vi "ActionVIOnCompile.vi"(8 "error in (no error)":errorcluster, 11 "Device Item Ref in":T2 format="%.0x") -> (0 "error out":errorcluster)   [LabVIEW 2015, in "SLSC Module Template System Explorer.lvlib"]
uses:
  SLSC Module Template System Explorer.lvlib
  <vilib>/NI Veristand/Custom Device API/Custom Device Item Ref.ctl
  Shared/SLSC Dynamic Channel.ctl
  Shared/Compiled.Settings
  Shared/Constants.vi
  <vilib>/NI Veristand/Custom Device Tools/Custom Device Utility Library/NI VeriStand - Search for Item by Name.vi
  <vilib>/NI Veristand/Custom Device API/Get Item Property (I32).vi
  <vilib>/NI Veristand/Custom Device API/Get Item Property (String).vi
  <vilib>/NI Veristand/Custom Device API/Set Item Property (Variant).vi
  <vilib>/NI Veristand/Custom Device Tools/Custom Device Utility Library/Custom Device Utility Library.lvlib
  <vilib>/NI Veristand/Custom Device API/Custom Device API.lvlib
  <vilib>/NI/NIVS Inline Async API/_Data Access System Explorer/Data Access System Explorer.lvlib
  Shared/SLSC Module Template Shared.lvlib
panel:
  out "SLSC Dynamic Commands":T1[](array[typedef])
  out "SLSC Dynamic outputs":T1[](array[typedef])
  out "SLSC Dynamic Inputs":T1[](array[typedef])
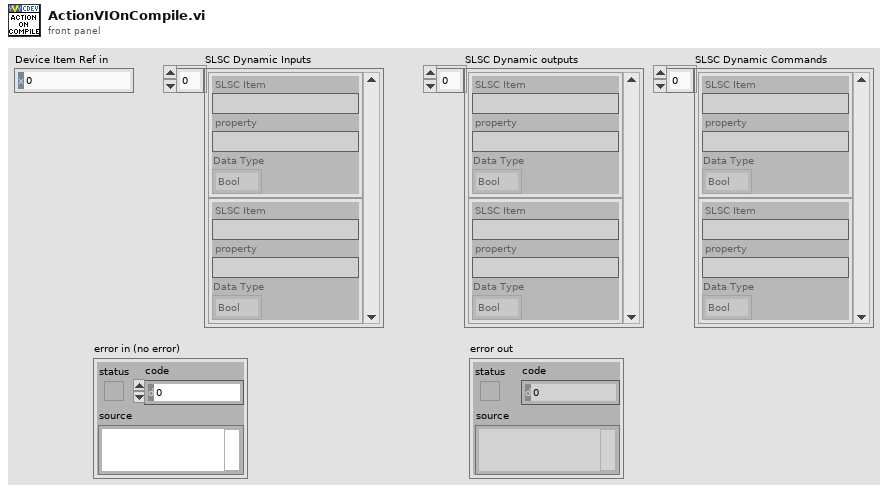
[diagram p1: front panel]
types:
  T1 = typedef "SLSC Module Template System Explorer.lvlib/SLSC Dynamic Channel.ctl" = cluster{"SLSC Item":string, "property":string, "Data Type":enum16{"Bool", "Double", "I32", "I64", "String", "U32", "U64"}}
  T2 = typedef "Custom Device API.lvlib/Custom Device Item Ref.ctl" = u64
  T3 = enum16{"Output/Write", "Input/Read", "Input/ReadWrite"}
  T4 = typedef "SLSC Module Template Shared.lvlib/Compiled.Settings" = cluster{"Name":string, "SLSC IP Address":string, "Slot #":i32, "Configuration Data":cluster{"Properties":cluster{"Boolean Properties":cluster{"property":refnum<k21>, "Value":bool, "SLSC Item":refnum<k21>}[], "Double Properties":cluster{"property":refnum<k21>, "Double Write":dbl, "SLSC Item":refnum<k21>}[], "I32 Properties":cluster{"property":refnum<k21>, "Int32 Write":i32, "SLSC Item":refnum<k21>}[], "I64 Properties":cluster{"property":refnum<k21>, "Int64 Write":i64, "SLSC Item":refnum<k21>}[], "String Properties":cluster{"property":refnum<k21>, "String Write":string, "SLSC Item":refnum<k21>}[], "U32 Properties":cluster{"property":refnum<k21>, "UInt32 Write":u32, "SLSC Item":refnum<k21>}[], "U64 Properties":cluster{"property":refnum<k21>, "UInt64 Write":u64, "SLSC Item":refnum<k21>}[]}}, "SLSC Dynamic Inputs":T1[], "SLSC Dynamic Outputs":T1[], "SLSC Dynamic Commands":T1[]}
  T5 = cluster{"Name":string, "Type":enum16{"Output/Write", "Input/Read", "Input/ReadWrite"}, "VS Refs":T2[]}
  T6 = typedef "Custom Device API.lvlib/Custom Device Item Info.ctl" = cluster{"Name":string, "Is Channel":bool, "GUID":string, "Is Waveform":bool}
  T7 = cluster{"Properties":cluster{"Boolean Properties":cluster{"property":refnum<k21>, "Value":bool, "SLSC Item":refnum<k21>}[], "Double Properties":cluster{"property":refnum<k21>, "Double Write":dbl, "SLSC Item":refnum<k21>}[], "I32 Properties":cluster{"property":refnum<k21>, "Int32 Write":i32, "SLSC Item":refnum<k21>}[], "I64 Properties":cluster{"property":refnum<k21>, "Int64 Write":i64, "SLSC Item":refnum<k21>}[], "String Properties":cluster{"property":refnum<k21>, "String Write":string, "SLSC Item":refnum<k21>}[], "U32 Properties":cluster{"property":refnum<k21>, "UInt32 Write":u32, "SLSC Item":refnum<k21>}[], "U64 Properties":cluster{"property":refnum<k21>, "UInt64 Write":u64, "SLSC Item":refnum<k21>}[]}}
  T8 = cluster{"Name":string, "Type":enum16{"Output/Write", "Input/Read", "Input/ReadWrite"}, "VS Refs":T2[]}[]
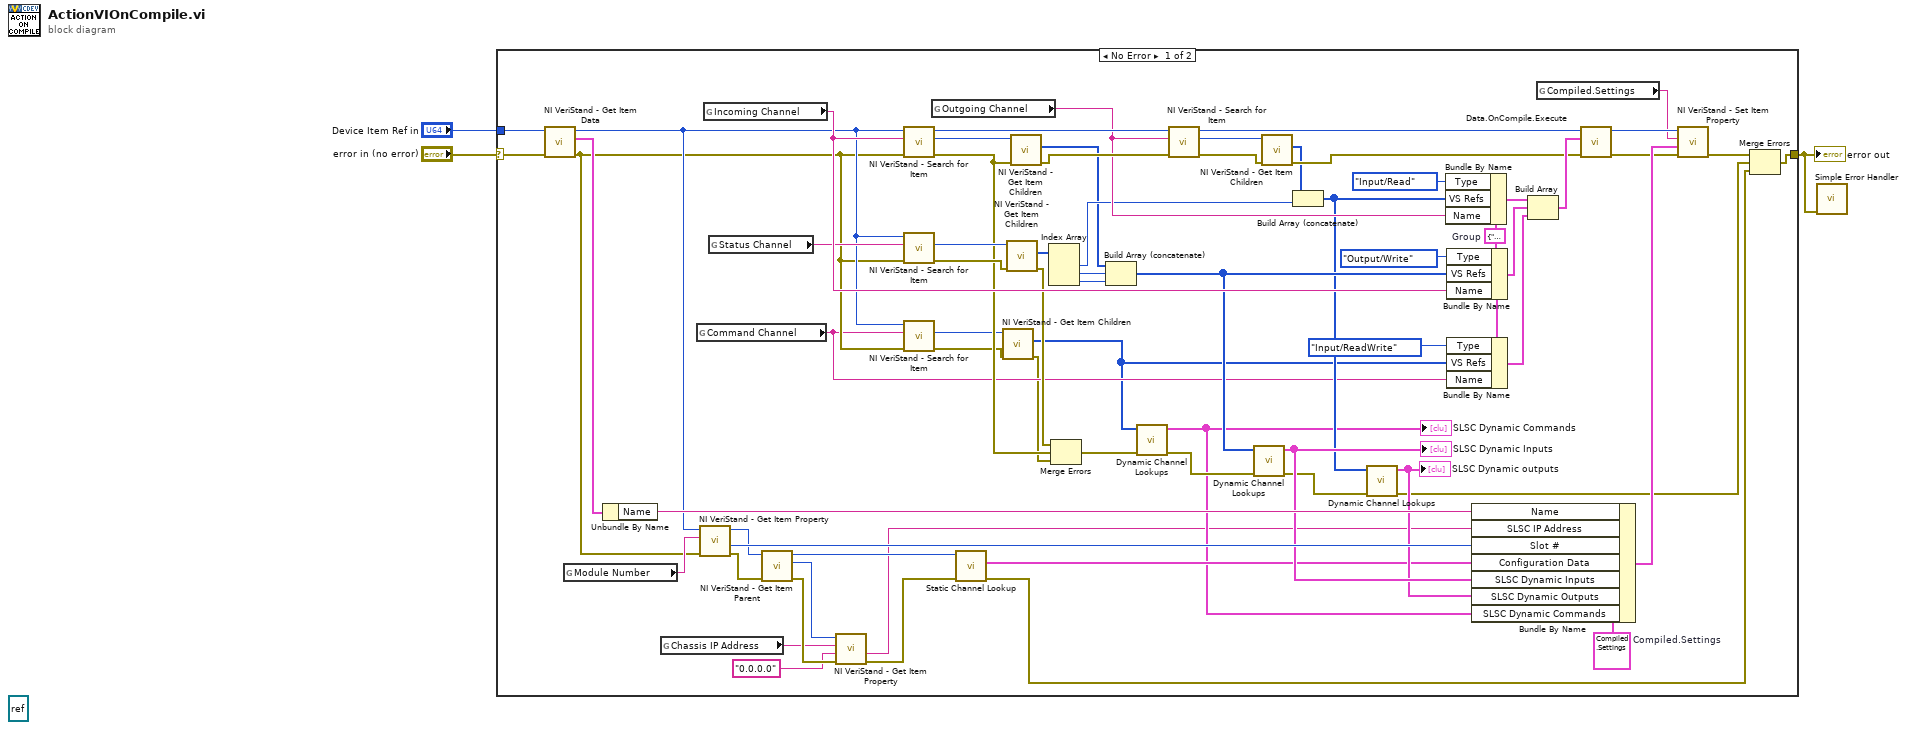
[diagram p0: block diagram]
diagram:
  (unwired) refnum<k7> refnum ("SHDocVw.IWebBrowser2")
  n1 = case shown="No Error" "error in (no error)" {
    selector: "error in (no error)" -> [w47 w72]
    tunnel: [w45 w72] -> w1
    tunnel: "Device Item Ref in" -> [w48 _]
    frame No Error {
      w38 = T4 {"Name"="", "SLSC IP Address"="", "Slot #"=0, "Configuration Data"={"Properties"={"Boolean Properties"=[], "Double Properties"=[], "I32 Properties"=[], "I64 Properties"=[], "String Properties"=[], "U32 Properties"=[], "U64 Properties"=[]}}, "SLSC Dynamic Inputs"=[], "SLSC Dynamic Outputs"=[], "SLSC Dynamic Commands"=[]}  # Compiled.Settings
      w12 = T5 {"Name"="", "Type"=enum."Output/Write", "VS Refs"=[]}  # Group
      n2 = call <vilib>:"NI VeriStand - Get Item Data.vi"("error in (no error)"=w47, "Item Ref in"=w48) -> ("error out"=w14:errorcluster, "Item Info"=w67:T6, "Item Ref out"=w15:T2)  [unwired: 6 in, 1 out]
      n3 = global read "Constants.vi" "Module Number"() -> (w50:string)
      n4 = Unbundle By Name(w67) -> ("Name"=w66:string)
      n5 = global read "Constants.vi" "Chassis IP Address"() -> (w49:string)
      n6 = global read "Constants.vi" "Command Channel"() -> (w13:string)
      n7 = call-poly <vilib>:"NI VeriStand - Get Item Property.vi"("error in (no error)"=w14, "Property Name"=w50, "Item Ref in"=w15) -> ("error out"=w54:errorcluster, "Value"=w51:i32, "Item Ref out"=w36:T2)  [unwired: 5 in, 1 out]
      n8 = global read "Constants.vi" "Incoming Channel"() -> (w41:string)
      n9 = global read "Constants.vi" "Status Channel"() -> (w27:string)
      n10 = call <vilib>:"NI VeriStand - Get Item Parent.vi"("error in (no error)"=w54, "Item Ref in"=w36) -> ("error out"=w53:errorcluster, "Parent Ref"=w52:T2, "Item Ref out"=w34:T2)  [unwired: 6 in, 1 out]
      n11 = call-poly <vilib>:"NI VeriStand - Get Item Property.vi"("error in (no error)"=w53, "Default Value"="0.0.0.0", "Property Name"=w49, "Item Ref in"=w52) -> ("error out"=w35:errorcluster, "Value"=w5:string)  [unwired: 4 in, 2 out]
      n12 = call-poly <vilib>:"NI VeriStand - Search for Item.vi"("error in"=w14, "Item Name"=w41, "Section Ref in"=w15) -> ("error out"=w21:errorcluster, "Item Ref"=w71:T2, "Section Ref out"=w58:T2)  [unwired: 5 in, 1 out]
      n13 = call-poly <vilib>:"NI VeriStand - Search for Item.vi"("error in"=w14, "Item Name"=w27, "Section Ref in"=w15) -> ("error out"=w32:errorcluster, "Item Ref"=w31:T2)  [unwired: 5 in, 2 out]
      n14 = call-poly <vilib>:"NI VeriStand - Search for Item.vi"("error in"=w14, "Item Name"=w13, "Section Ref in"=w15) -> ("error out"=w17:errorcluster, "Item Ref"=w18:T2)  [unwired: 5 in, 2 out]
      n15 = global read "Constants.vi" "Outgoing Channel"() -> (w40:string)
      n16 = call "Static Channel Lookup.vi"("error in (no error)"=w35, "Device Item Ref in"=w34) -> ("error out"=w19:errorcluster, "Configuration Data"=w37:T7)  [unwired: 7 in, 1 out]
      n17 = call <vilib>:"NI VeriStand - Get Item Children.vi"("error in (no error)"=w17, "Item Ref in"=w18) -> ("error out"=w11:errorcluster, "Child Refs"=w7:T2[])  [unwired: 6 in, 2 out]
      n18 = call <vilib>:"NI VeriStand - Get Item Children.vi"("error in (no error)"=w32, "Item Ref in"=w31) -> ("error out"=w20:errorcluster, "Child Refs"=w28:T2[])  [unwired: 6 in, 2 out]
      n19 = call <vilib>:"NI VeriStand - Get Item Children.vi"("error in (no error)"=w21, "Item Ref in"=w71) -> ("error out"=w57:errorcluster, "Child Refs"=w22:T2[])  [unwired: 6 in, 2 out]
      n20 = Index Array(array=w28) -> (element #1=w23:T2, element #2=w30:T2, element #3=w29:T2)  [unwired: 3 in]
      n21 = Merge Errors(w20, w21, w11) -> (w9:errorcluster)
      n22 = Build Array (concatenate)(w22, w30, w29) -> (w26:T2[])
      n23 = call "Dynamic Channel Lookups.vi"("error in (no error)"=w9, "Child Refs"=w7) -> ("error out"=w8:errorcluster, "SLSC Dynamic Inputs"=w6:T1[])  [unwired: 8 in]
      "SLSC Dynamic Commands" <- w6
      n24 = call-poly <vilib>:"NI VeriStand - Search for Item.vi"("error in"=w57, "Item Name"=w40, "Section Ref in"=w58) -> ("error out"=w43:errorcluster, "Item Ref"=w70:T2, "Section Ref out"=w59:T2)  [unwired: 5 in, 1 out]
      n25 = call "Dynamic Channel Lookups.vi"("error in (no error)"=w8, "Child Refs"=w26) -> ("error out"=w42:errorcluster, "SLSC Dynamic Inputs"=w44:T1[])  [unwired: 8 in]
      "SLSC Dynamic Inputs" <- w44
      n26 = call <vilib>:"NI VeriStand - Get Item Children.vi"("error in (no error)"=w43, "Item Ref in"=w70) -> ("error out"=w60:errorcluster, "Child Refs"=w24:T2[])  [unwired: 6 in, 2 out]
      n27 = Build Array (concatenate)(w24, w23) -> (w25:T2[])
      n28 = call "Dynamic Channel Lookups.vi"("error in (no error)"=w42, "Child Refs"=w25) -> ("error out"=w33:errorcluster, "SLSC Dynamic Inputs"=w39:T1[])  [unwired: 8 in]
      "SLSC Dynamic outputs" <- w39
      n29 = Bundle By Name(cluster=w12, "Type"=T3."Input/Read", "VS Refs"=w25, "Name"=w40) -> (w65:T5)
      n30 = Bundle By Name(cluster=w12, "Type"=T3."Output/Write", "VS Refs"=w26, "Name"=w41) -> (w61:T5)
      n31 = Bundle By Name(cluster=w12, "Type"=T3."Input/ReadWrite", "VS Refs"=w7, "Name"=w13) -> (w10:T5)
      n32 = Bundle By Name(cluster=w38, "Name"=w66, "SLSC IP Address"=w5, "Slot #"=w51, "Configuration Data"=w37, "SLSC Dynamic Inputs"=w44, "SLSC Dynamic Outputs"=w39, "SLSC Dynamic Commands"=w6) -> (w69:T4)
      n33 = Build Array(w65, w61, w10) -> (w63:T8)
      n34 = global read "Constants.vi" "Compiled.Settings"() -> (w46:string)
      n35 = call <vilib>:"Data.OnCompile.Execute.vi"("error in"=w60, "VS Ref Groups"=w63, "Custom Device Ref"=w59) -> ("error out"=w56:errorcluster, "Custom Device Ref"=w55:T2)  [unwired: 7 in]
      n36 = call-poly <vilib>:"NI VeriStand - Set Item Property.vi"("error in (no error)"=w56, "Value"=w69, "Property Name"=w46, "Item Ref in"=w55) -> ("error out"=w68:errorcluster)  [unwired: 5 in, 2 out]
      n37 = Merge Errors(w68, w33, w19) -> (w45:errorcluster)
    }
    frame Error {
    }
  }
  "error out" <- w1
  n38 = call <vilib>:"Simple Error Handler.vi"("error in (no error)"=w1) -> ()  [unwired: 4 in, 5 out]
